vi "Initialize.vi"(8 "error in (no error)":errorcluster, 10 "Device":string, 11 "Thermocouple in":refnum<class "Thermocouple.lvclass">) -> (0 "error out":errorcluster, 3 "Thermocouple out":refnum<class "Thermocouple.lvclass">)   [LabVIEW 2018, in "Thermocouple.lvlib" / "Thermocouple.lvclass"]
uses:
  Thermocouple.lvclass
  Thermocouple.lvclass/Thermocouple.ctl
  PPLs/Utilities/Configuration.lvlibp/Configuration.lvclass
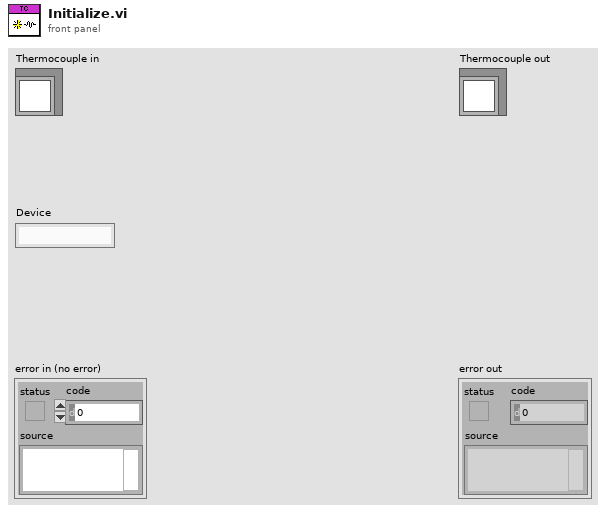
[diagram p1: front panel]
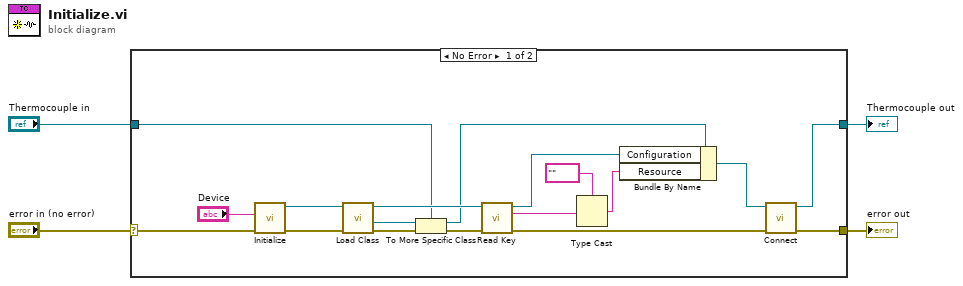
[diagram p0: block diagram]
diagram:
  n1 = case shown="No Error" "error in (no error)" {
    selector: "error in (no error)" -> [w21 w24]
    tunnel: [w7 w24] -> w3
    tunnel: [w9 w23] -> w1
    tunnel: "Thermocouple in" -> [w10 w23]
    frame No Error {
      n2 = call "Initialize.vi"("error in"=w21, "Device"="Device") -> ("error out"=w19:errorcluster, "Configuration out"=w20:refnum<class "Configuration.lvclass">)  [unwired: 8 in]
      n3 = call "Load Class.vi"("error in"=w19, "Configuration in"=w20) -> ("error out"=w18:errorcluster, "Class out"=w17:refnum<class>, "Configuration out"=w16:refnum<class "Configuration.lvclass">)  [unwired: 7 in]
      n4 = To More Specific Class(target class=w10, reference=w17, error in=w18) -> (specific class reference=w14:refnum<class "Thermocouple.lvclass">, error out=w15:errorcluster)
      n5 = call "Read Key.vi"("error in"=w15, "Configuration in"=w16) -> ("error out"=w8:errorcluster, "Value"=w12:string, "Configuration out"=w13:refnum<class "Configuration.lvclass">)  [unwired: 7 in]
      n6 = Type Cast(type=tag "" ("Resource"), x=w12) -> (*(type *) &x=w5:tag)
      n7 = Bundle By Name(cluster=w14, "Configuration"=w13, "Resource"=w5) -> (w11:refnum<class "Thermocouple.lvclass">)
      n8 = call-dynamic "Connect.vi"("error in (no error)"=w8, "Thermocouple in"=w11) -> ("error out"=w7:errorcluster, "Thermocouple out"=w9:refnum<class "Thermocouple.lvclass">)  [unwired: 8 in]
    }
    frame Error {
    }
  }
  "error out" <- w3
  "Thermocouple out" <- w1
